vi "Write Source Mode.vi"(8 "error in (no error)":errorcluster, 10 "Source Mode":T1, 11 "Power Supply in":refnum<class "Power Supply.lvclass">) -> (0 "error out":errorcluster, 3 "Power Supply out":refnum<class "Power Supply.lvclass">)   [LabVIEW 2011, in "Power Supply.lvclass"]
uses:
  Power Supply.lvclass
  Source Mode.ctl
  Power Supply.lvclass/Power Supply.ctl
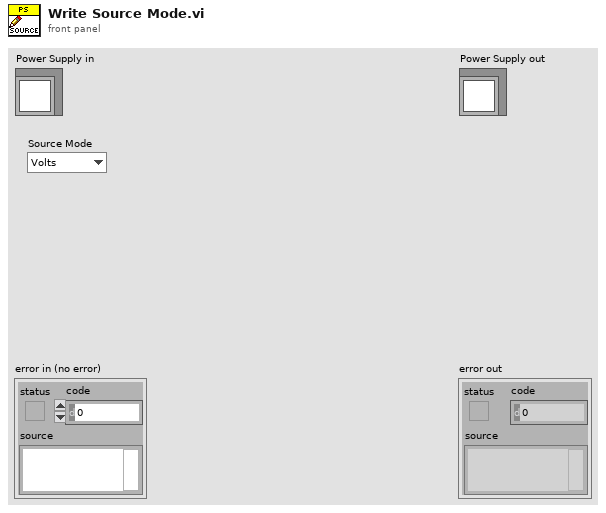
[diagram p1: front panel]
types:
  T1 = typedef "Power Supply.lvclass/Source Mode.ctl" = enum16{"Volts", "Current"}
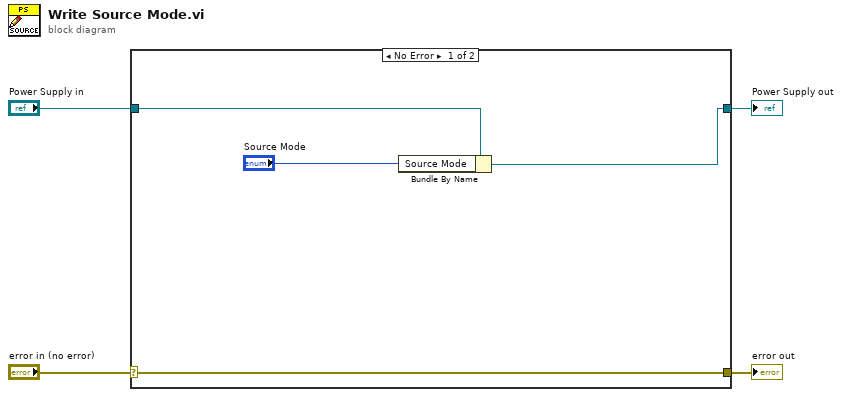
[diagram p0: block diagram]
diagram:
  n1 = case shown="No Error" "error in (no error)" {
    selector: "error in (no error)" -> [w8 w10]
    tunnel: [w8 w10] -> w3
    tunnel: [w5 w9] -> w1
    tunnel: "Power Supply in" -> [w7 w9]
    frame No Error {
      n2 = Bundle By Name(cluster=w7, "Source Mode"="Source Mode") -> (w5:refnum<class "Power Supply.lvclass">)
    }
    frame Error {
    }
  }
  "error out" <- w3
  "Power Supply out" <- w1
